vi "f_5_Tr.vi"(0 "file path (IN)":path, 1 "Project #":string, 2 "Request #":string, 3 "TEST #":string, 5 "error in (no error)":errorcluster, 6 "ICE":dbl) -> (11 "Di (A)":dbl, 13 "Dt (ns)":dbl, 14 "file path (OUT)":path, 15 "Tr (ns)":dbl, 16 "Di/Dt (A/us)":dbl, 17 "DONE Tr":bool, 18 "DONE Di/Dt ON":bool, 19 "error out":errorcluster)   [LabVIEW 2020]
uses:
  GlobIndSw1.vi
  <vilib>/Waveform/WDTOps.llb/WDT Waveform Duration DBL.vi
  <vilib>/Waveform/WDTOps.llb/WDT Get Waveform Subset DBL.vi
  <vilib>/measure/mamon.llb/Trigger Detection for 1 Channel.vi
  <vilib>/Analysis/NI_AALBase.lvlib
  <vilib>/measure/NI_MAPro.lvlib
panel:
  in  "Decision ?":bool
  out "Dt (us)":dbl
  out "90% Ice":dbl
  out "10% Ice":dbl
  out "Cursor a : Channel 1":dbl
  out "Cursor b : Channel 1":dbl
  out "Waveform Graph":waveform(dbl)[](graph)
  out "ON Region":waveform(dbl)[](graph) caption="Tr (ns) & DiDt on (A/us)"
  # "Tr = from 10% Ice to 90% Ice"
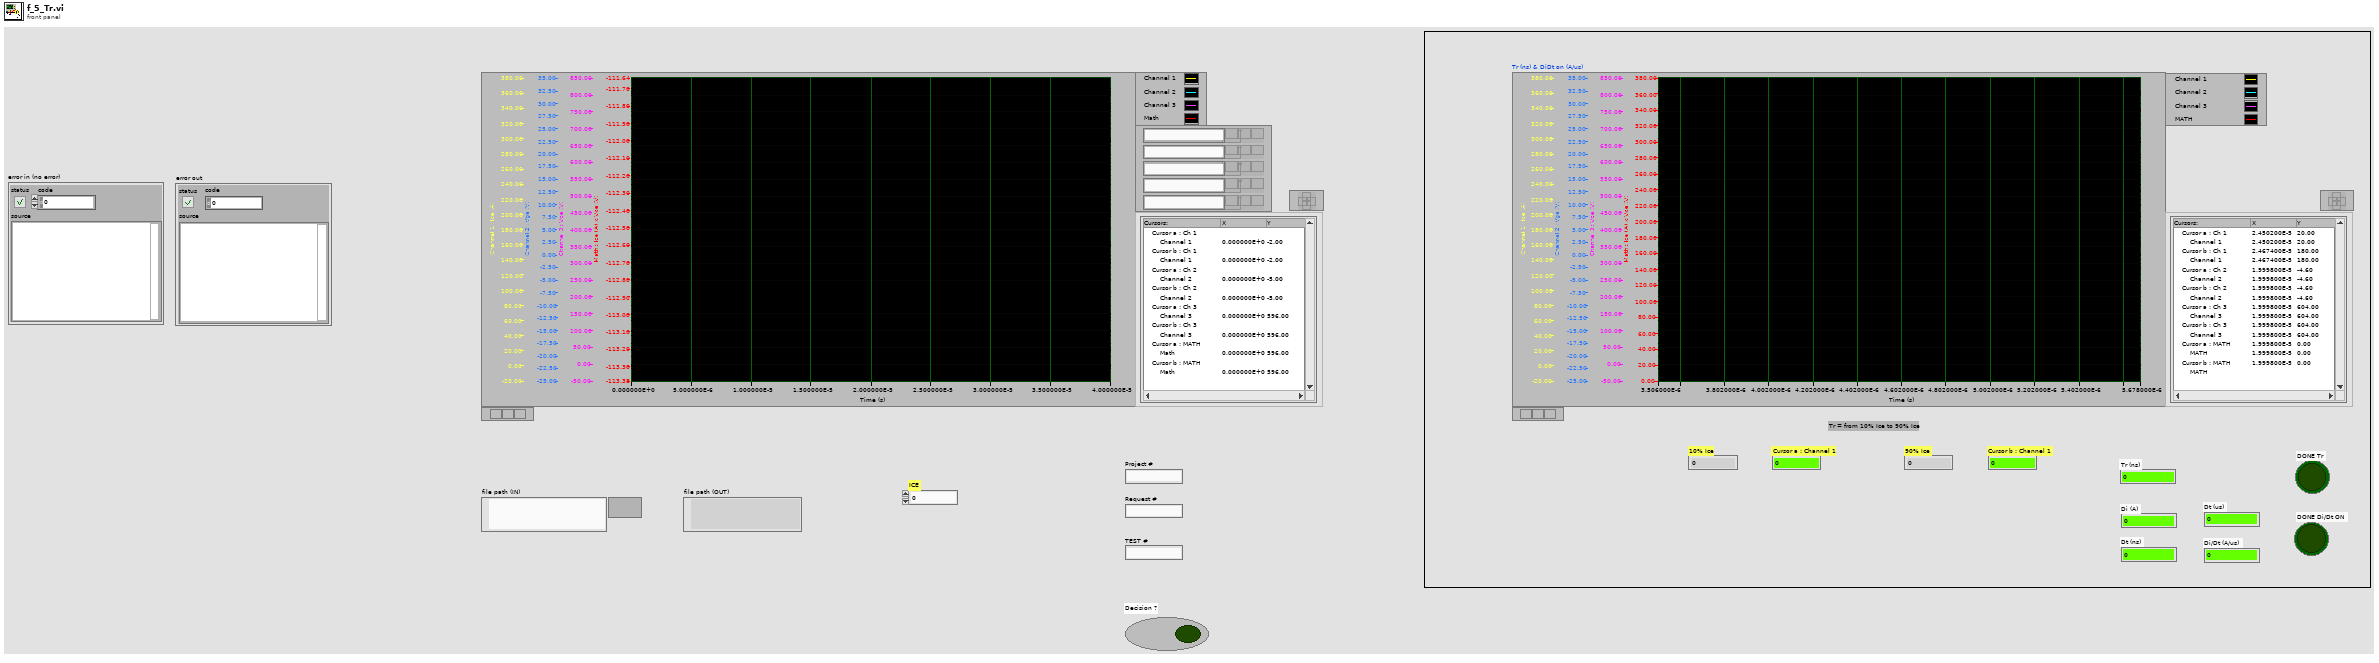
[diagram p1: front panel]
types:
  T1 = enum32{"Invalid", "Standard", "Closed", "Hidden", "Minimized", "Maximized"}
  T2 = typedef "imagedata.ctl" = cluster{"image type":i32, "image depth":i32, "image":u8[], "mask":u8[], "colors":u32[], "Rectangle":cluster{"left":i16, "top":i16, "right":i16, "bottom":i16}}
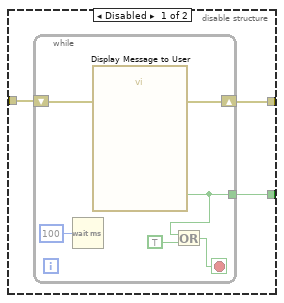
[diagram p2: hidden frame]
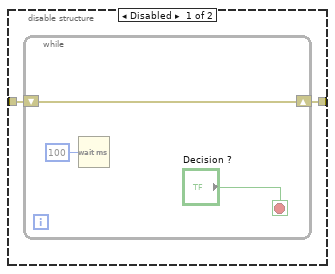
[diagram p7: hidden frame]
diagram:
  w2 = FALSE ("DONE Tdon")
  w1 = 0.0 ("Cursor a : Channel 1")
  w3 = errorcluster {"status"=FALSE, "code"=0, "source"=""} ("error out")
  w4 = waveform(dbl)[] [] ("Waveform Graph")
  n1 = disable-structure shown="Disabled" {
    frame Disabled {
      n2 = control-ref of="This VI"() -> (w11:refnum<vi>)
      n3 = control-ref of="This VI"() -> (w12:refnum<vi>)
      n4 = invoke class="VI" method="FP.Close"(reference=w11) -> ()  [unwired: 2 in, 3 out]
      n5 = invoke class="VI" method="FP.Open"(reference=w12, "Activate"=TRUE ("Activate?"), "State"=T1."Maximized") -> (error in=w15:errorcluster, error out=w13:errorcluster)  [unwired: 1 in, 4 out]
      n6 = property class="VI"(reference=w12, error in=w13, "Front Panel.Closeable"=TRUE ("Front Panel Window:Closeable")) -> ()  [unwired: 2 out]
    }
    frame Enabled {
    }
  }
  n7 = local write "Cursor a : Channel 1"(w1) -> ()
  n8 = local write "Cursor b : Channel 1"(w1) -> ()
  n9 = local write "DONE Di/Dt ON"(w2) -> ()
  n10 = local write "Decision ?"(w2) -> ()
  n11 = local write "DONE Tr"(w2) -> ()
  n12 = local write "Tr (ns)"(w1) -> ()
  n13 = local write "Di (A)"(w1) -> ()
  n14 = local write "Dt (ns)"(w1) -> ()
  n15 = local write "Dt (us)"(w1) -> ()
  n16 = local write "Di/Dt (A/us)"(w1) -> ()
  n17 = local write "error out"(w3) -> ()
  n18 = local write "error in (no error)"(w3) -> ()
  n19 = local write "Waveform Graph"(w4) -> ()
  n20 = local write "ON Region"(w4) -> ()
  n21 = flat-sequence {
    tunnel: ["file path (IN)"] -> w10
    tunnel: [w18] -> w9
    tunnel: [w27] -> w8
    tunnel: [w26] -> w7
    tunnel: w10 -> [w29]
    tunnel: w9 -> [w28]
    tunnel: [w285] -> w6
    tunnel: w8 -> [w284]
    tunnel: w7 -> [w283]
    tunnel: [w283] -> w5
    tunnel: w6 -> [w300]
    tunnel: w5 -> [w299]
    frame #0 {
      n22 = control-ref of="This VI"() -> (w23:refnum<vi>)
      n23 = invoke class="VI" method="FP.Open"(reference=w23, error in="error in (no error)", "Activate"=TRUE ("Activate?"), "State"=T1."Maximized") -> (error out=w24:errorcluster)  [unwired: 1 in, 4 out]
      n24 = property class="VI"(reference=w23, error in=w24, "Front Panel.Closeable"=TRUE ("Front Panel Window:Closeable")) -> (error out=w18:errorcluster)  [unwired: 1 out]
    }
    frame #1 {
      n25 = while {
        tunnel: w29 -> [w37]
        shift-right: [w32] -> w27
        shift-left: w28 -> [w36]
        tunnel: [w34] -> w26
        stop <- w31 stop-if-true
        n26 = flat-sequence {
          tunnel: [w71] -> w55
          tunnel: [w72] -> w54
          tunnel: w37 -> [w72]
          tunnel: w36 -> [w71]
          tunnel: w55 -> [w168]
          tunnel: w54 -> [w162]
          tunnel: [w93] -> w53
          tunnel: [w83] -> w52
          tunnel: [w74] -> w30
          tunnel: w53 -> [w212]
          tunnel: [w222] -> w51
          tunnel: w52 -> [w231]
          tunnel: [w231] -> w50
          tunnel: [w218] -> w49
          tunnel: [w221] -> w48
          tunnel: [w203] -> w47
          tunnel: [w213] -> w46
          tunnel: w30 -> [w206]
          tunnel: w51 -> [w252]
          tunnel: [w251] -> w45
          tunnel: w50 -> [w253]
          tunnel: [w253] -> w44
          tunnel: w49 -> [w246]
          tunnel: [w246] -> w43
          tunnel: w48 -> [w245]
          tunnel: [w245] -> w42
          tunnel: w47 -> [w243]
          tunnel: [w243] -> w41
          tunnel: w46 -> [w244]
          tunnel: [w244] -> w40
          tunnel: w45 -> [w255]
          tunnel: w44 -> [w268]
          tunnel: [w268] -> w39
          tunnel: w43 -> [w262]
          tunnel: w42 -> [w263]
          tunnel: w41 -> [w261]
          tunnel: w40 -> [w260]
          tunnel: [w255] -> w38
          tunnel: w39 -> [w273]
          tunnel: w38 -> [w275]
          tunnel: [w274] -> w33
          tunnel: [w273] -> w34
          frame #0 {
            w68 = waveform(dbl)[] [] ("Waveform Graph")
            w67 = 0.0 ("Cursor a : Channel 1")
            w70 = FALSE ("DONE Tdon")
            n27 = local write "Cursor a : Channel 1"(w67) -> ()
            n28 = local write "Cursor b : Channel 1"(w67) -> ()
            n29 = local write "DONE Di/Dt ON"(w70) -> ()
            n30 = local write "Decision ?"(w70) -> ()
            n31 = local write "DONE Tr"(w70) -> ()
            n32 = local write "Tr (ns)"(w67) -> ()
            n33 = local write "Di (A)"(w67) -> ()
            n34 = local write "Dt (ns)"(w67) -> ()
            n35 = local write "Dt (us)"(w67) -> ()
            n36 = local write "Di/Dt (A/us)"(w67) -> ()
            n37 = Wait (ms)(milliseconds to wait=u32 300) -> ()  [unwired: 1 out]
            n38 = local write "Waveform Graph"(w68) -> ()
            n39 = local write "ON Region"(w68) -> ()
          }
          frame #1 {
            w143 = u16 1 items=["Samples", "Relative Time"] ("start/duration format")
            w154 = u16 1 items=["Samples", "Relative Time"] ("start/duration format")
            w155 = u16 1 items=["Samples", "Relative Time"] ("start/duration format")
            # "Channel 1"
            # "Channel 3"
            # "Channel 2"
            # "dt"
            # "Ch2"
            # "Ch1"
            n40 = call "3_ReadDatatoWaveform.vi"("error in (no error)"=w168, "file path (IN)"=w162) -> ("error out"=w76:errorcluster, "Waveform Graph"=→"Waveform Graph":waveform(dbl)[], "file path (OUT)"=w83:path, "dt"=w163:dbl, "Ch 2 Data"=w160:dbl[], "Ch 3 Data"=w164:dbl[], "Ch 1 Data"=w161:dbl[])  [unwired: 3 in]
            n41 = Wait (ms)(milliseconds to wait=u32 400) -> ()  [unwired: 1 out]
            n42 = call <vilib>:"Beep.vi"("use system alert? (T)"=FALSE, "duration (msec)"=u32 200, "frequency (Hz)"=u32 2000) -> ()  [unwired: 9 in]
            n43 = To Time Stamp(1:0.0 ("number")) -> (0:w165:timestamp)
            n44 = disable-structure shown="Enabled" {
              disable-tunnel: w165 -> [w187 _]
              disable-tunnel: w163 -> [w186 _]
              disable-tunnel: w161 -> [w185 _]
              disable-tunnel: [w184 _] -> w78
              frame Enabled {
                # "Channel 1"
                n45 = Bundle By Name("Y"=w185, "dt"=w186, "t0"=w187) -> (w184:waveform(dbl))  [unwired: 1 in]
              }
              frame Disabled {
              }
            }
            n46 = disable-structure shown="Enabled" {
              disable-tunnel: w165 -> [w191 _]
              disable-tunnel: w163 -> [w190 _]
              disable-tunnel: w160 -> [w189 _]
              disable-tunnel: [w188 _] -> w142
              frame Enabled {
                # "Channel 2"
                n47 = Bundle By Name("Y"=w189, "dt"=w190, "t0"=w191) -> (w188:waveform(dbl))  [unwired: 1 in]
              }
              frame Disabled {
              }
            }
            n48 = disable-structure shown="Enabled" {
              disable-tunnel: w165 -> [w195 _]
              disable-tunnel: w163 -> [w194 _]
              disable-tunnel: w164 -> [w193 _]
              disable-tunnel: [w192 _] -> w141
              frame Enabled {
                # "Channel 3"
                n49 = Bundle By Name("Y"=w193, "dt"=w194, "t0"=w195) -> (w192:waveform(dbl))  [unwired: 1 in]
              }
              frame Disabled {
              }
            }
            n50 = disable-structure shown="Enabled" {
              disable-tunnel: w78 -> [w180 _]
              disable-tunnel: [w172 _] -> w79
              disable-tunnel: [w171 _] -> w74
              disable-tunnel: w76 -> [w170 _]
              frame Enabled {
                w174 = u16 1 items=["Samples", "Relative Time"] ("start/duration format")
                # "Channel 1 - Filtered"
                # "Median"
                n51 = global read "GlobIndSw1.vi" "Median Filter Rank"() -> (w169:i32)
                n52 = Unbundle By Name(w180) -> ("Y"=w183:dbl[], "dt"=w181:dbl)
                n53 = call <vilib>:"Median Filter.vi"("right rank"=w169, "left rank"=w169, "X"=w183) -> ("Filtered X"=w182:dbl[])  [unwired: 7 in, 1 out]
                n54 = Bundle By Name("Y"=w182, "dt"=w181) -> (w173:waveform(dbl))  [unwired: 1 in]
                n55 = call-poly <vilib>:"Waveform Duration.vi"("error in (no error)"=w170, "waveform in"=w173) -> ("error out"=w177:errorcluster, "duration"=w179:dbl, "waveform out"=w178:waveform(dbl))  [unwired: 7 in]
                n56 = Divide(x=w179, y=2.0) -> (x/y=w176:dbl)
                n57 = call-poly <vilib>:"Get Waveform Subset.vi"("start/duration format"=w174, "error in (no error)"=w177, "duration"=w176, "start samples/time"=w176, "waveform in"=w178) -> ("error out"=w172:errorcluster, "waveform out"=w171:waveform(dbl))  [unwired: 1 in, 2 out]
              }
              frame Disabled {
              }
            }
            n58 = call-poly <vilib>:"Waveform Duration.vi"("error in (no error)"=w76, "waveform in"=w78) -> ("error out"=w159:errorcluster, "duration"=w156:dbl, "waveform out"=w158:waveform(dbl))  [unwired: 7 in]
            n59 = call-poly <vilib>:"Waveform Duration.vi"("error in (no error)"=w76, "waveform in"=w142) -> ("error out"=w149:errorcluster, "duration"=w152:dbl, "waveform out"=w150:waveform(dbl))  [unwired: 7 in]
            n60 = call-poly <vilib>:"Waveform Duration.vi"("error in (no error)"=w76, "waveform in"=w141) -> ("error out"=w148:errorcluster, "duration"=w145:dbl, "waveform out"=w147:waveform(dbl))  [unwired: 7 in]
            n61 = Divide(x=w156, y=2.0) -> (x/y=w138:dbl)
            n62 = Divide(x=w152, y=2.0) -> (x/y=w153:dbl)
            n63 = Divide(x=w145, y=2.0) -> (x/y=w144:dbl)
            n64 = call-poly <vilib>:"Get Waveform Subset.vi"("start/duration format"=w155, "error in (no error)"=w159, "duration"=w138, "start samples/time"=w138, "waveform in"=w158) -> ("error out"=w137:errorcluster, "waveform out"=w94:waveform(dbl))  [unwired: 1 in, 2 out]
            n65 = call-poly <vilib>:"Get Waveform Subset.vi"("start/duration format"=w154, "error in (no error)"=w149, "duration"=w153, "start samples/time"=w153, "waveform in"=w150) -> ("error out"=w136:errorcluster, "waveform out"=w95:waveform(dbl))  [unwired: 1 in, 2 out]
            n66 = call-poly <vilib>:"Get Waveform Subset.vi"("start/duration format"=w143, "error in (no error)"=w148, "duration"=w144, "start samples/time"=w144, "waveform in"=w147) -> ("error out"=w75:errorcluster, "waveform out"=w140:waveform(dbl))  [unwired: 1 in, 2 out]
            n67 = Build Array(w94, w95, w140, waveform(dbl) {"t0"=timestamp(0 s since 1904-01-01), "dt"=1.0, "Y"=[]} ("element")) -> (→"ON Region":waveform(dbl)[])
            n68 = Merge Errors(w137, w136, w75, w79) -> (w91:errorcluster)
            n69 = property on="ON Region" class="WFGraph (strict)"(error in=w91) -> (error out=w90:errorcluster, "Width"=w89:u32)  [unwired: 1 in, 1 out]
            n70 = property on="ON Region" class="WFGraph (strict)"(error in=w90, "Caption.Justify"=enum16{"Left", "Center", "Right"}."Left" ("Caption.Justification"), "Caption.Width"=w89, "Caption.FontBold"=TRUE ("Caption.Font:Bold"), "Caption.FontColor"=u32 16860 ("Caption.Font:Color"), "Caption.FontSize"=u32 24 ("Caption.Font:Size"), "Caption.Text"="Tr (ns) & DiDt on (A/us)") -> (error out=w85:errorcluster)  [unwired: 1 in, 1 out]
            n71 = property on="ON Region" class="WFGraph (strict)"(error in=w85, "XScale.Offset"=w138) -> (error out=w119:errorcluster)  [unwired: 1 in, 1 out]
            n72 = property on="ON Region" class="WFGraph (strict)"(error in=w119, "Active Cursor"=u32 0, "Cursor.Cursor X"=0.0 ("Cursor.Cursor Position:Cursor X"), "Cursor.Cursor Y"=0.0 ("Cursor.Cursor Position:Cursor Y"), "Cursor.Visible"=FALSE) -> (error out=w118:errorcluster)  [unwired: 1 in, 1 out]
            n73 = property on="ON Region" class="WFGraph (strict)"(error in=w118, "Active Cursor"=u32 1, "Cursor.Cursor X"=0.0 ("Cursor.Cursor Position:Cursor X"), "Cursor.Cursor Y"=0.0 ("Cursor.Cursor Position:Cursor Y"), "Cursor.Visible"=FALSE) -> (error out=w117:errorcluster)  [unwired: 1 in, 1 out]
            n74 = property on="ON Region" class="WFGraph (strict)"(error in=w117, "Active Cursor"=u32 2, "Cursor.Cursor X"=0.0 ("Cursor.Cursor Position:Cursor X"), "Cursor.Cursor Y"=0.0 ("Cursor.Cursor Position:Cursor Y"), "Cursor.Visible"=FALSE) -> (error out=w116:errorcluster)  [unwired: 1 in, 1 out]
            n75 = property on="ON Region" class="WFGraph (strict)"(error in=w116, "Active Cursor"=u32 3, "Cursor.Cursor X"=0.0 ("Cursor.Cursor Position:Cursor X"), "Cursor.Cursor Y"=0.0 ("Cursor.Cursor Position:Cursor Y"), "Cursor.Visible"=FALSE) -> (error out=w99:errorcluster)  [unwired: 1 in, 1 out]
            n76 = property on="ON Region" class="WFGraph (strict)"(error in=w99, "Active Cursor"=u32 4, "Cursor.Cursor X"=0.0 ("Cursor.Cursor Position:Cursor X"), "Cursor.Cursor Y"=0.0 ("Cursor.Cursor Position:Cursor Y"), "Cursor.Visible"=FALSE) -> (error out=w98:errorcluster)  [unwired: 1 in, 1 out]
            n77 = property on="ON Region" class="WFGraph (strict)"(error in=w98, "Active Cursor"=u32 5, "Cursor.Cursor X"=0.0 ("Cursor.Cursor Position:Cursor X"), "Cursor.Cursor Y"=0.0 ("Cursor.Cursor Position:Cursor Y"), "Cursor.Visible"=FALSE) -> (error out=w97:errorcluster)  [unwired: 1 in, 1 out]
            n78 = property on="ON Region" class="WFGraph (strict)"(error in=w97, "Active Cursor"=u32 6, "Cursor.Cursor X"=0.0 ("Cursor.Cursor Position:Cursor X"), "Cursor.Cursor Y"=0.0 ("Cursor.Cursor Position:Cursor Y"), "Cursor.Visible"=FALSE) -> (error out=w96:errorcluster)  [unwired: 1 in, 1 out]
            n79 = property on="ON Region" class="WFGraph (strict)"(error in=w96, "Active Cursor"=u32 7, "Cursor.Cursor X"=0.0 ("Cursor.Cursor Position:Cursor X"), "Cursor.Cursor Y"=0.0 ("Cursor.Cursor Position:Cursor Y"), "Cursor.Visible"=FALSE) -> (error out=w93:errorcluster)  [unwired: 1 in, 1 out]
          }
          frame #2 {
            w209 = u16 1 items=["Falling Edge", "Rising Edge"] ("trigger slope")
            w210 = u16 1 items=["Index", "Time"] ("location mode")
            w216 = u16 1 items=["Falling Edge", "Rising Edge"] ("trigger slope")
            w217 = u16 1 items=["Index", "Time"] ("location mode")
            # "Cursor a : Channel 1"
            # "Cursor b : Channel 1"
            # "Cursor b : Channel 1"
            # "Cursor a : Channel 1"
            # "Cursor b : Channel 1"
            # "Cursor a : Channel 1"
            # "Cursor b : Channel 1"
            # "Cursor a : Channel 1"
            # "End Time 1st Cursor"
            # "End Time 2nd Cursor"
            # "1st PARAMETER : 10% Ice"
            # "Channel 1"
            # "2nd PARAMETER : 90% Ice"
            # "Channel 1"
            n80 = Divide(x=10.0, y=100.0) -> (x/y=w241:dbl)
            n81 = Wait (ms)(milliseconds to wait=u32 500) -> ()  [unwired: 1 out]
            n82 = Multiply(x=w241, y="ICE") -> (x*y=w214:dbl)
            "10% Ice" <- w214
            n83 = Add(x=w214, y=0.2) -> (x+y=w201:dbl)
            n84 = Divide(x=w201, y=10.0) -> (x/y=w200:dbl)
            n85 = call <vilib>:"Beep.vi"("use system alert? (T)"=FALSE, "duration (msec)"=u32 200, "frequency (Hz)"=u32 2000) -> ()  [unwired: 9 in]
            n86 = call-poly <vilib>:"Basic Level Trigger Detection.vi"("signal in"=w206, "level"=w201, "hysteresis"=w200, "location mode"=w217, "error in (no error)"=w212, "trigger slope"=w216) -> ("trigger location"=w213:dbl, "error out"=w211:errorcluster)  [unwired: 7 in, 1 out]
            n87 = property on="ON Region" class="WFGraph (strict)"(error in=w211, "Active Cursor"=u32 0, "Cursor.Cursor X"=w213, "Cursor.Visible"=TRUE, "Cursor.Cursor Name Visible"=TRUE) -> (error out=w226:errorcluster)  [unwired: 1 in, 1 out]
            n88 = property on="ON Region" class="WFGraph (strict)"(error in=w226, "Active Cursor"=u32 0) -> (error out=w205:errorcluster, "Cursor.Cursor Y"=w218:dbl)  [unwired: 1 in, 1 out]
            "Cursor a : Channel 1" <- w218
            n89 = Divide(x=90.0, y=100.0) -> (x/y=w238:dbl)
            n90 = Multiply(x=w238, y="ICE") -> (x*y=w207:dbl)
            "90% Ice" <- w207
            n91 = Add(x=w207, y=0.2) -> (x+y=w198:dbl)
            n92 = Divide(x=w198, y=10.0) -> (x/y=w197:dbl)
            n93 = call-poly <vilib>:"Basic Level Trigger Detection.vi"("signal in"=w206, "level"=w198, "hysteresis"=w197, "location mode"=w210, "error in (no error)"=w205, "trigger slope"=w209) -> ("trigger location"=w203:dbl, "error out"=w204:errorcluster)  [unwired: 7 in, 1 out]
            n94 = property on="ON Region" class="WFGraph (strict)"(error in=w204, "Active Cursor"=u32 1, "Cursor.Cursor X"=w203, "Cursor.Visible"=TRUE, "Cursor.Cursor Name Visible"=TRUE) -> (error out=w223:errorcluster)  [unwired: 1 in, 1 out]
            n95 = property on="ON Region" class="WFGraph (strict)"(error in=w223, "Active Cursor"=u32 1) -> (error out=w222:errorcluster, "Cursor.Cursor Y"=w221:dbl)  [unwired: 1 in, 1 out]
            "Cursor b : Channel 1" <- w221
          }
          frame #3 {
            # "2nd Cursor"
            # "1st Cursor"
            n96 = Subtract(x=w244, y=1e-06) -> (x-y=w247:dbl)
            n97 = Add(x=w243, y=1e-06) -> (x+y=w248:dbl)
            n98 = property on="ON Region" class="WFGraph (strict)"(error in=w252, "XScale.Minimum"=w247, "XScale.Maximum"=w248) -> (error out=w251:errorcluster)  [unwired: 1 in, 1 out]
            n99 = Wait (ms)(milliseconds to wait=u32 300) -> ()  [unwired: 1 out]
          }
          frame #4 {
            # "us"
            # "ns"
            n100 = Subtract(x=w263, y=w262) -> (x-y=w258:dbl)
            n101 = Subtract(x=w261, y=w260) -> (x-y=w259:dbl)
            n102 = Absolute Value(x=w258) -> (abs(x)=w257:dbl)
            "Di (A)" <- w257
            n103 = Absolute Value(x=w259) -> (abs(x)=w256:dbl)
            n104 = Multiply(x=w256, y=1000000000.0) -> (x*y=→"Tr (ns)" →"Dt (ns)":dbl)
            n105 = Multiply(x=w256, y=1000000.0) -> (x*y=w265:dbl)
            "Dt (us)" <- w265
            n106 = Wait (ms)(milliseconds to wait=u32 300) -> ()  [unwired: 1 out]
            n107 = call <vilib>:"Beep.vi"("use system alert? (T)"=FALSE, "duration (msec)"=u32 200, "frequency (Hz)"=u32 2000) -> ()  [unwired: 9 in]
            n108 = Divide(x=w257, y=w265) -> (x/y=→"Di/Dt (A/us)":dbl)
          }
          frame #5 {
            n109 = disable-structure shown="Enabled" {
              disable-tunnel: w275 -> [w277 w281]
              disable-tunnel: [w276 w281] -> w274
              frame Disabled {
                n110 = while {
                  shift-right: [w278] -> w276
                  shift-left: w277 -> [w278]
                  stop <- "Decision ?" stop-if-true
                  n111 = Wait (ms)(milliseconds to wait=u32 100) -> ()  [unwired: 1 out]
                }
              }
              frame Enabled {
              }
            }
          }
        }
        n112 = disable-structure shown="Enabled" {
          disable-tunnel: w33 -> [w58 w65]
          disable-tunnel: [w57 w65] -> w32
          disable-tunnel: [w56 TRUE ("NO")] -> w31
          frame Disabled {
            n113 = while {
              tunnel: [w60] -> w56
              shift-right: [w63] -> w57
              shift-left: w58 -> [w64]
              stop <- w62 stop-if-true
              n114 = Wait (ms)(milliseconds to wait=u32 100) -> ()  [unwired: 1 out]
              n115 = call "Display Message to User"("error in (no error)"=w64) -> ("error out"=w63:errorcluster, "NO"=w60:bool)  [unwired: 9 in]
              n116 = Or(x=w60, y=TRUE) -> (x .or. y?=w62:bool)
            }
          }
          frame Enabled {
          }
        }
        n117 = Wait (ms)(milliseconds to wait=u32 100) -> ()  [unwired: 1 out]
      }
    }
    frame #2 {
      w288 = "_"
      n118 = Wait (ms)(milliseconds to wait=u32 300) -> ()  [unwired: 1 out]
      n119 = invoke on="ON Region" class="WFGraph (strict)" method="Get Image"(error in=w284) -> (error out=w292:errorcluster, "image data"=w295:T2)  [unwired: 5 in, 4 out]
      n120 = Concatenate Strings("C:\\Inductive_Switching_Project\\IndSw_Image\\" ("string"), "Project #", w288, "Request #", w288, "TEST #", w288, "Tr_DiDton" ("string"), ".png" ("string")) -> (w296:string)
      n121 = String To Path(string=w296) -> (path=w294:path)
      n122 = call <vilib>:"Write PNG File.vi"("error in (no error)"=w292, "image data"=w295, "path to PNG file"=w294) -> ("error out"=w285:errorcluster)  [unwired: 7 in, 1 out]
      "DONE Tr" <- TRUE ("DONE Tdon")
      "DONE Di/Dt ON" <- TRUE ("DONE Di/Dt ON")
    }
    frame #3 {
      n123 = disable-structure shown="Enabled" {
        disable-tunnel: w300 -> [w301 _]
        frame Enabled {
          n124 = control-ref of="This VI"() -> (w302:refnum<vi>)
          n125 = invoke class="VI" method="FP.Close"(reference=w302, error in=w301) -> ()  [unwired: 1 in, 3 out]
        }
        frame Disabled {
        }
      }
      "error out" <- w300
      "file path (OUT)" <- w299
    }
  }
